vi "Read Font.vi"(8 "error in":errorcluster, 11 "Font in":refnum<k24>) -> (0 "error out":errorcluster, 2 "Font":T1={"Bold"=enum."bold", "Italic"=enum."italic", "Underline"=enum."double", "TextColor"=242688, "TextSize"=18.0, "Name"="Calibri"}, 3 "Font out":refnum<k24>)   [LabVIEW 2019, in "Open Xml.lvlib"]
uses:
  Open Xml.lvlib
  D:/git/Open-Xml-LabVIEW/Source/DocumentFormat.OpenXml.dll
  DocumentFormat.OpenXml.dll
  D:/git/Open-Xml-LabVIEW/Source/DocumentFormat.OpenXml.Framework.dll
  DocumentFormat.OpenXml.Framework.dll
  Font.ctl
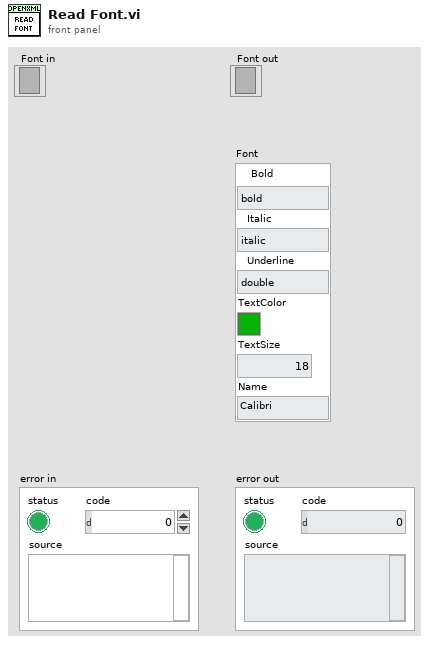
[diagram p1: front panel]
types:
  T1 = typedef "Open Xml.lvlib/Font.ctl" = cluster{"Bold":enum16{"bold", "regular", "default"}, "Italic":enum16{"italic", "regular", "default"}, "Underline":enum16{"single", "double", "singleAccounting", "doubleAccounting", "none", "default"}, "TextColor":u32, "TextSize":dbl, "Name":string}
  T2 = enum16{"single", "double", "singleAccounting", "doubleAccounting", "none", "default"}
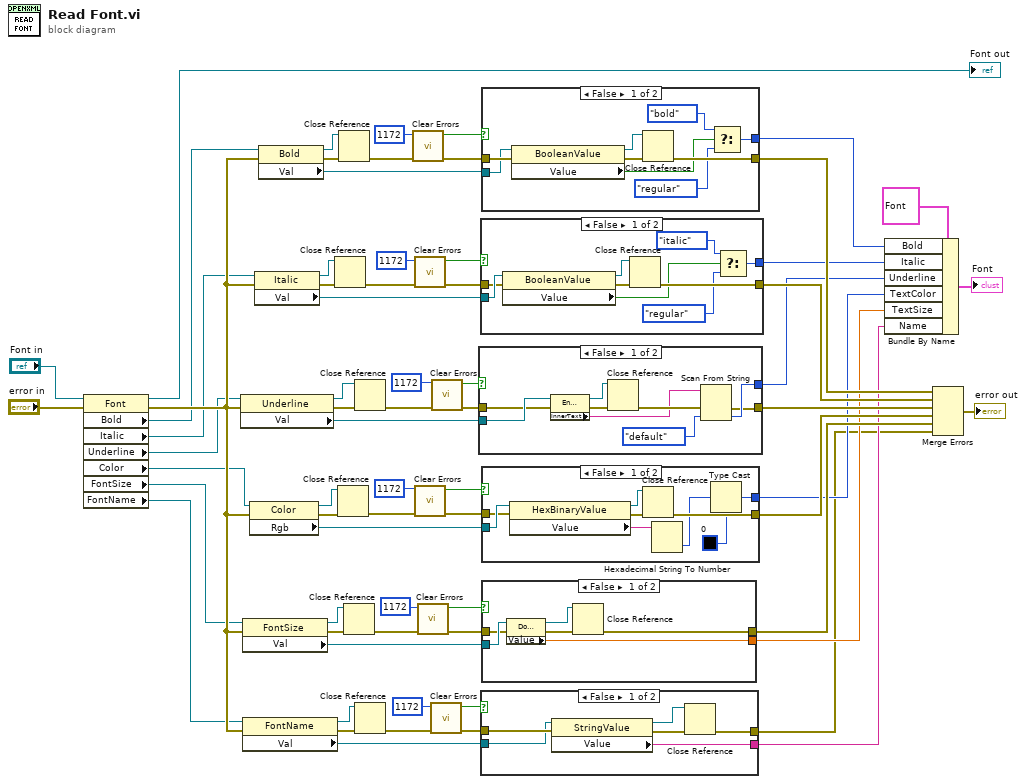
[diagram p0: block diagram]
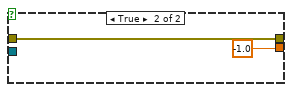
[diagram p3: hidden frame]
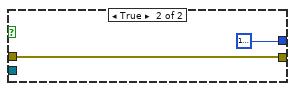
[diagram p4: hidden frame]
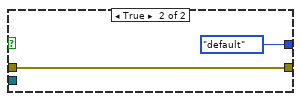
[diagram p5: hidden frame]
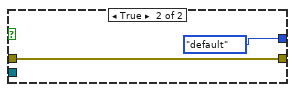
[diagram p6: hidden frame]
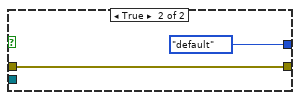
[diagram p7: hidden frame]
diagram:
  n1 = property class="Font"(reference="Font in", error in="error in") -> (reference out=→"Font out":refnum<k24>, error out=w50:errorcluster, "Bold"=w42:refnum<k24>, "Italic"=w43:refnum<k24>, "Underline"=w44:refnum<k24>, "Color"=w45:refnum<k24>, "FontSize"=w46:refnum<k24>, "FontName"=w47:refnum<k24>)
  n2 = property class="Underline"(reference=w44, error in=w50) -> (reference out=w25:refnum<k24>, error out=w55:errorcluster, "Val"=w56:refnum<k24>)
  n3 = property class="FontSize"(reference=w46, error in=w50) -> (reference out=w11:refnum<k24>, error out=w57:errorcluster, "Val"=w49:refnum<k24>)
  n4 = property class="FontName"(reference=w47, error in=w50) -> (reference out=w58:refnum<k24>, error out=w59:errorcluster, "Val"=w1:refnum<k24>)
  n5 = property class="Color"(reference=w45, error in=w50) -> (reference out=w17:refnum<k24>, error out=w18:errorcluster, "Rgb"=w48:refnum<k24>)
  n6 = property class="Italic"(reference=w43, error in=w50) -> (reference out=w36:refnum<k24>, error out=w54:errorcluster, "Val"=w53:refnum<k24>)
  n7 = property class="Bold"(reference=w42, error in=w50) -> (reference out=w31:refnum<k24>, error out=w52:errorcluster, "Val"=w51:refnum<k24>)
  n8 = Close Reference(reference=w36, error in (no error)=w54) -> (error out=w37:errorcluster)
  n9 = Close Reference(reference=w17, error in (no error)=w18) -> (error out=w20:errorcluster)
  n10 = Close Reference(reference=w31, error in (no error)=w52) -> (error out=w32:errorcluster)
  n11 = Close Reference(reference=w11, error in (no error)=w57) -> (error out=w12:errorcluster)
  n12 = Close Reference(reference=w25, error in (no error)=w55) -> (error out=w26:errorcluster)
  n13 = Close Reference(reference=w58, error in (no error)=w59) -> (error out=w65:errorcluster)
  n14 = call <vilib>:"Clear Errors.vi"("error in (no error)"=w32, "specific error code to clear (0: all)"=1172) -> ("error out"=w30:errorcluster, "specific error cleared?"=w28:bool)  [unwired: 4 in]
  n15 = call <vilib>:"Clear Errors.vi"("error in (no error)"=w37, "specific error code to clear (0: all)"=1172) -> ("error out"=w39:errorcluster, "specific error cleared?"=w35:bool)  [unwired: 4 in]
  n16 = call <vilib>:"Clear Errors.vi"("error in (no error)"=w20, "specific error code to clear (0: all)"=1172) -> ("error out"=w15:errorcluster, "specific error cleared?"=w16:bool)  [unwired: 4 in]
  n17 = call <vilib>:"Clear Errors.vi"("error in (no error)"=w12, "specific error code to clear (0: all)"=1172) -> ("error out"=w10:errorcluster, "specific error cleared?"=w8:bool)  [unwired: 4 in]
  n18 = call <vilib>:"Clear Errors.vi"("error in (no error)"=w65, "specific error code to clear (0: all)"=1172) -> ("error out"=w4:errorcluster, "specific error cleared?"=w2:bool)  [unwired: 4 in]
  n19 = call <vilib>:"Clear Errors.vi"("error in (no error)"=w26, "specific error code to clear (0: all)"=1172) -> ("error out"=w24:errorcluster, "specific error cleared?"=w22:bool)  [unwired: 4 in]
  n20 = case shown="False" w22 {
    tunnel: [w69 w77] -> w62
    tunnel: w56 -> [w74 _]
    tunnel: w24 -> [w73 w77]
    tunnel: [w71 T2."default" ("Underline")] -> w21
    frame False {
      n21 = property class="EnumValue`1[[DocumentFormat.Ope"(reference=w74, error in=w73) -> (reference out=w75:refnum<k24>, error out=w76:errorcluster, "InnerText"=w68:string)
      n22 = Close Reference(reference=w75, error in (no error)=w76) -> (error out=w70:errorcluster)
      n23 = Scan From String(input string=w68, error in=w70, default 1=T2."default" ("Underline")) -> (error out=w69:errorcluster, output 1=w71:T2)  [unwired: 2 in, 2 out]
    }
    frame True {
    }
  }
  n24 = case shown="False" w35 {
    tunnel: [w87 w89] -> w61
    tunnel: w53 -> [w84 _]
    tunnel: w39 -> [w83 w89]
    tunnel: [w81 enum16{"italic", "regular", "default"}."default" ("Italic")] -> w33
    frame False {
      n25 = property class="BooleanValue"(reference=w84, error in=w83) -> (reference out=w85:refnum<k24>, error out=w86:errorcluster, "Value"=w82:bool)
      n26 = Close Reference(reference=w85, error in (no error)=w86) -> (error out=w87:errorcluster)
      n27 = Select(t=enum16{"italic", "regular", "default"}."italic" ("Italic"), s=w82, f=enum16{"italic", "regular", "default"}."regular" ("Italic")) -> (s? t:f=w81:enum16{"italic", "regular", "default"})
    }
    frame True {
    }
  }
  n28 = case shown="False" w2 {
    tunnel: [w90 _] -> w5
    tunnel: w4 -> [w95 w96]
    tunnel: [w93 w96] -> w3
    tunnel: w1 -> [w91 _]
    frame False {
      n29 = property class="StringValue"(reference=w91, error in=w95) -> (reference out=w92:refnum<k24>, error out=w94:errorcluster, "Value"=w90:string)
      n30 = Close Reference(reference=w92, error in (no error)=w94) -> (error out=w93:errorcluster)
    }
    frame True {
    }
  }
  n31 = case shown="False" w28 {
    tunnel: [w105 w107] -> w60
    tunnel: w30 -> [w102 w107]
    tunnel: w51 -> [w101 _]
    tunnel: [w100 enum16{"bold", "regular", "default"}."default" ("Bold")] -> w27
    frame False {
      n32 = property class="BooleanValue"(reference=w101, error in=w102) -> (reference out=w103:refnum<k24>, error out=w104:errorcluster, "Value"=w98:bool)
      n33 = Close Reference(reference=w103, error in (no error)=w104) -> (error out=w105:errorcluster)
      n34 = Select(t=enum16{"bold", "regular", "default"}."bold" ("Bold"), s=w98, f=enum16{"bold", "regular", "default"}."regular") -> (s? t:f=w100:enum16{"bold", "regular", "default"})
    }
    frame True {
    }
  }
  n35 = case shown="False" w16 {
    tunnel: [w116 w118] -> w63
    tunnel: w48 -> [w113 _]
    tunnel: w15 -> [w112 w118]
    tunnel: [w110 u32 16777216 ("Color")] -> w14
    frame False {
      n36 = property class="HexBinaryValue"(reference=w113, error in=w112) -> (reference out=w115:refnum<k24>, error out=w114:errorcluster, "Value"=w109:string)
      n37 = Close Reference(reference=w115, error in (no error)=w114) -> (error out=w116:errorcluster)
      n38 = Hexadecimal String To Number(string=w109) -> (number=w108:u32)  [unwired: 2 in, 1 out]
      n39 = Type Cast(type=u32 0 ("Color"), x=w108) -> (*(type *) &x=w110:u32)
    }
    frame True {
    }
  }
  n40 = case shown="False" w8 {
    tunnel: [w124 w126] -> w64
    tunnel: w49 -> [w121 _]
    tunnel: w10 -> [w120 w126]
    tunnel: [w119 -1.0 ("Value")] -> w7
    frame False {
      n41 = property class="DoubleValue"(reference=w121, error in=w120) -> (reference out=w122:refnum<k24>, error out=w123:errorcluster, "Value"=w119:dbl)
      n42 = Close Reference(reference=w122, error in (no error)=w123) -> (error out=w124:errorcluster)
    }
    frame True {
    }
  }
  n43 = Bundle By Name(cluster=T1 {"Bold"=enum."bold", "Italic"=enum."italic", "Underline"=enum."double", "TextColor"=242688, "TextSize"=18.0, "Name"="Calibri"} ("Font"), "Bold"=w27, "Italic"=w33, "Underline"=w21, "TextColor"=w14, "TextSize"=w7, "Name"=w5) -> (→"Font":T1)
  n44 = Merge Errors(w60, w61, w62, w63, w64, w3) -> (→"error out":errorcluster)
